vi "Destination Lat Long Given Distance.vi"(9 "Bearing (clockwise from North)":dbl, 10 "Distance (km)":dbl, 11 "Origin Point":T1 {"Y Coordinate" format="%#_10g"; "X Coordinate" format="%#_10g"}) -> (3 "Destination Point":T1 {"Y Coordinate" format="%#_10g"; "X Coordinate" format="%#_10g"})   [LabVIEW 2014]
uses:
  Control/SHX Point Data.ctl
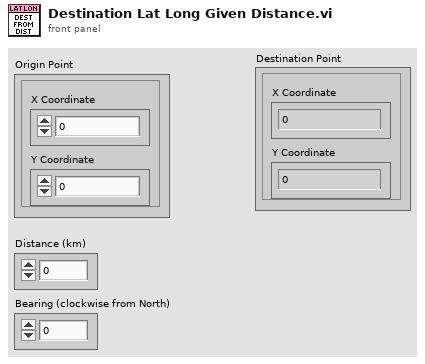
[diagram p1: front panel]
types:
  T1 = typedef "SHX Point Data.ctl" = cluster{"X Coordinate":dbl, "Y Coordinate":dbl}
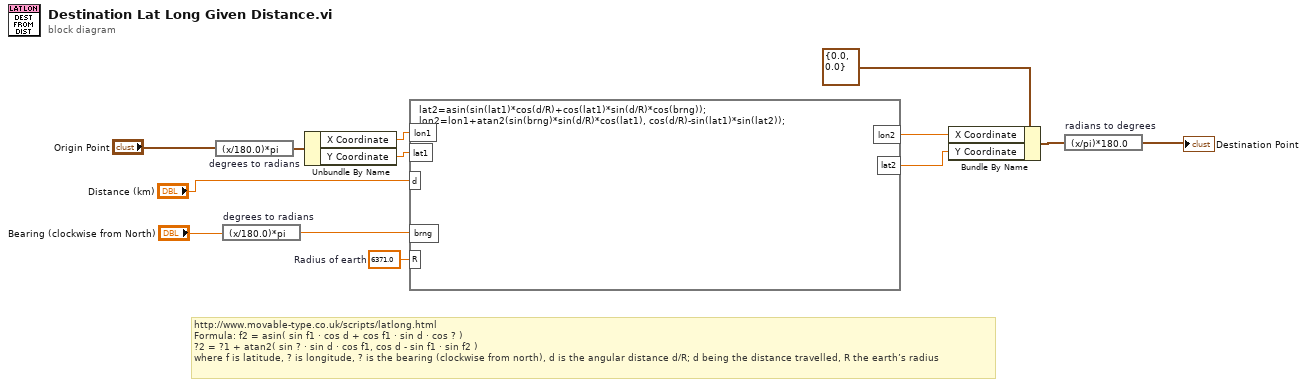
[diagram p0: block diagram]
diagram:
  w7 = 6371.0  # Radius of earth
  # "http://www.movable-type.co.uk/scripts/latlong.html\nFormula:\tf2 = asin( sin f1 · cos d + cos f1 · sin d · cos ? )\n?2 = ?1 + atan2( sin ? · sin d · cos f1, cos d - sin f1 · sin f2 )\nwhere\tf is latitude, ? is longitude, ? is the bearing (clockwise from north), d is the angular distance d/R; d being the distance travelled, R the earth’s radius"
  n1 = expression code="(x/180.0)*pi" "degrees to radians"("Origin Point") -> (w12:T1)
  n2 = expression code="(x/180.0)*pi" "degrees to radians"("Bearing (clockwise from North)") -> (w8:dbl)
  n3 = Unbundle By Name(w12) -> ("X Coordinate"=w10:dbl, "Y Coordinate"=w11:dbl)
  n4 = formula code="lat2=asin(sin(lat1)*cos(d/R)+cos(lat1)*sin(d/R)*cos(brng));\nlon2=lon1+atan2(sin(brng)*sin(d/R)*cos(lat1), cos(d/R)-sin(lat1)*sin(lat2));"("lon1"=w10, "lat1"=w11, "brng"=w8, "d"="Distance (km)", "R"=w7) -> ("lat2"=w4:dbl, "lon2"=w5:dbl)
  n5 = Bundle By Name(cluster=T1 {"X Coordinate"=0.0, "Y Coordinate"=0.0} ("SHX Point"), "X Coordinate"=w5, "Y Coordinate"=w4) -> (w3:T1)
  n6 = expression code="(x/pi)*180.0" "radians to degrees"(w3) -> (→"Destination Point":T1)
